vi "StringMergerProj1.vi"(0 "Username":string, 5 "PartType":string, 7 "Min Voltage":dbl, 9 "Max Voltage":dbl, 11 "Step":dbl) -> (4 "Output string":string)   [LabVIEW 2021]
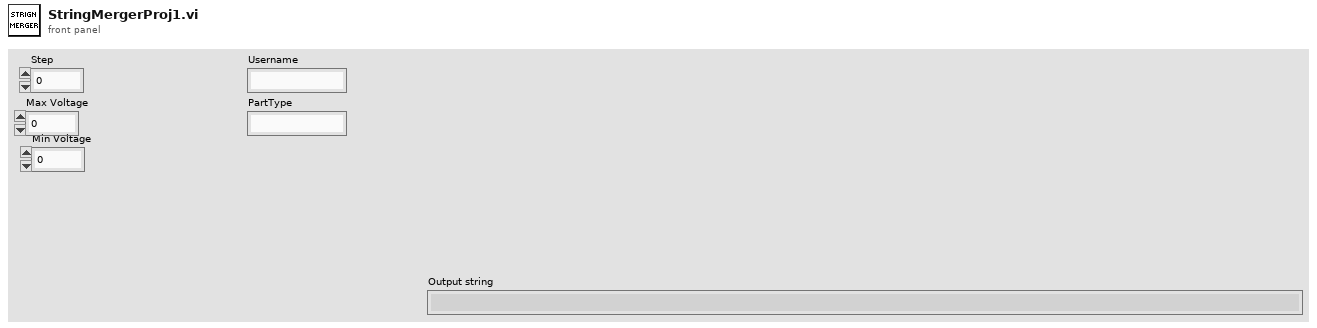
[diagram p1: front panel]
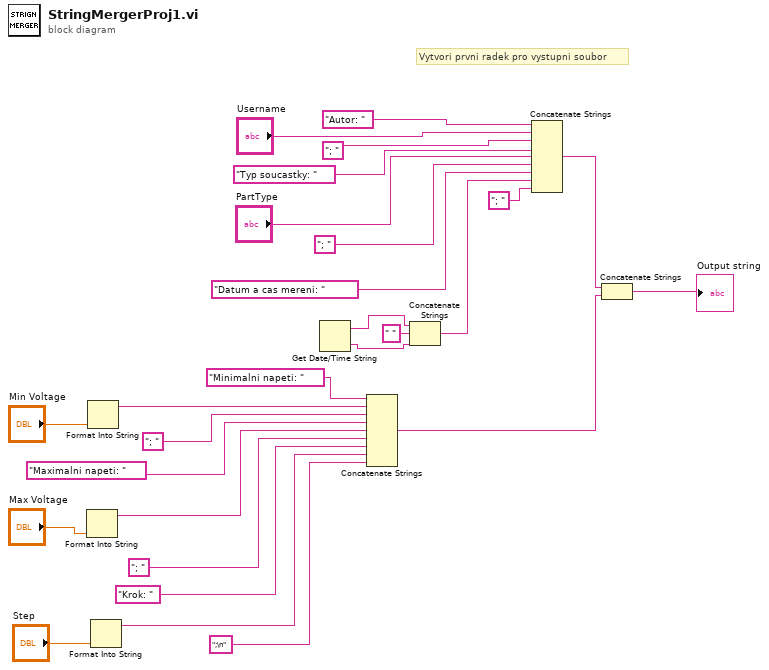
[diagram p0: block diagram]
diagram:
  # "Vytvori prvni radek pro vystupni soubor"
  n1 = Format Into String("Max Voltage") -> (resulting string=w3:string)  [unwired: 3 in, 1 out]
  n2 = Format Into String("Min Voltage") -> (resulting string=w6:string)  [unwired: 3 in, 1 out]
  n3 = Format Into String("Step") -> (resulting string=w1:string)  [unwired: 3 in, 1 out]
  n4 = Get Date/Time String() -> (date string=w19:string, time string=w18:string)  [unwired: 3 in]
  n5 = Concatenate Strings("Minimalni napeti: " ("string"), w6, "; " ("string"), "Maximalni napeti: " ("string"), w3, "; " ("string"), "Krok: " ("string"), w1, ";\n" ("string")) -> (w9:string)
  n6 = Concatenate Strings(w19, " " ("string"), w18) -> (w17:string)
  n7 = Concatenate Strings("Autor: " ("string"), "Username", "; " ("string"), "Typ soucastky: " ("string"), "PartType", "; " ("string"), "Datum a cas mereni: " ("string"), w17, "; " ("string")) -> (w8:string)
  n8 = Concatenate Strings(w8, w9) -> (→"Output string":string)
